vi "test.vi"() -> ()   [LabVIEW 2023]
uses:
  enum_kontrola.ctl
panel:
  in  "stop":bool
  out "Numeric":dbl
  in  "Enum":T1
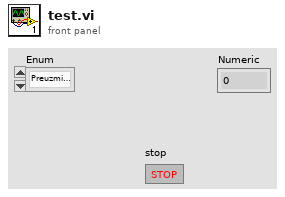
[diagram p1: front panel]
types:
  T1 = typedef "enum_kontrola.ctl" = enum16{"Preuzmi vrijednost", "Ponisti", "Povecaj", "Smanji"}
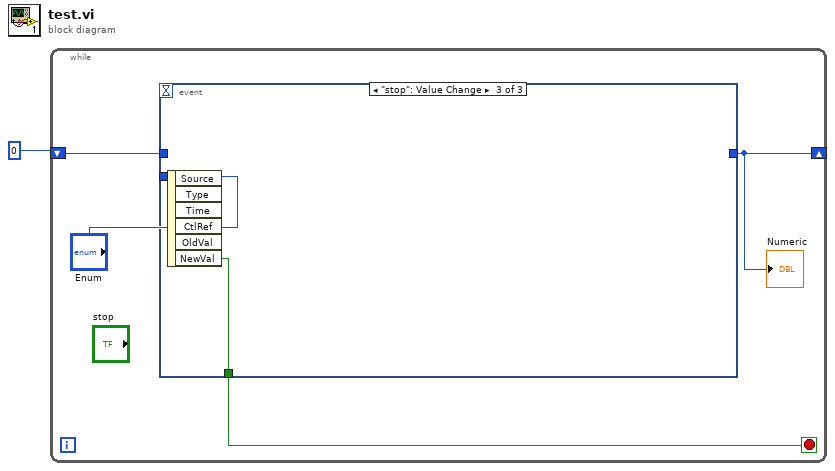
[diagram p0: block diagram]
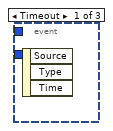
[diagram p2: hidden frame]
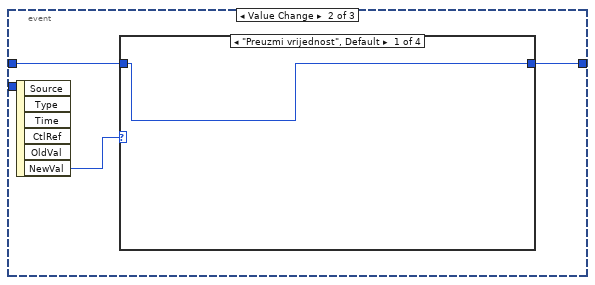
[diagram p3: hidden frame]
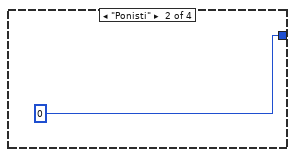
[diagram p4: hidden frame]
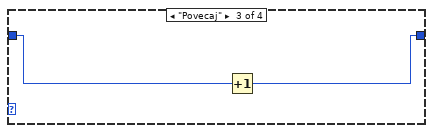
[diagram p5: hidden frame]
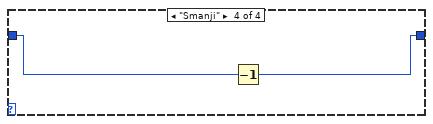
[diagram p6: hidden frame]
diagram:
  n1 = while {
    shift-right: [w3] -> _
    shift-left: 0 -> [w4]
    stop <- w2 stop-if-true
    n2 = event shown="[2] \"stop\": Value Change" {
      selector: _ -> [_ _ _]
      dyn-events: _ -> [_ _ _]
      timeout: _ -> [_ _ _]
      tunnel: "Enum" -> [_ _ _]
      tunnel: w4 -> [_ w7 _]
      tunnel: [_ w6 _] -> w3
      tunnel: [_ _ w15] -> w2
      event Timeout {
        n3 = event-data() -> ()  [unwired: 1 in, 3 out]
      }
      event Value Change {
        n4 = event-data() -> ("NewVal"=w8:T1)  [unwired: 1 in, 5 out]
        n5 = case shown="\"Preuzmi vrijednost\", Default" w8 {
          tunnel: w7 -> [w9 _ w11 w13]
          tunnel: [w9 0 w12 w14] -> w6
          frame "Preuzmi vrijednost", Default {
          }
          frame "Ponisti" {
          }
          frame "Povecaj" {
            n6 = Increment(x=w11) -> (x+1=w12:i32)
          }
          frame "Smanji" {
            n7 = Decrement(x=w13) -> (x-1=w14:i32)
          }
        }
      }
      event "stop": Value Change {
        n8 = event-data() -> ("NewVal"=w15:bool)  [unwired: 1 in, 5 out]
      }
    }
    "Numeric" <- w3
  }
